vi "FindValueFromParameterNameList.vi"(10 "String":string, 11 "Matlab Param Data":T1[](array[typedef])) -> (2 "found?":bool, 3 "Matlab Data Bundle":T1)   [LabVIEW 2017]
uses:
  Types/MatlabDataBundle.ctl
  Types/MatlabDataType.ctl
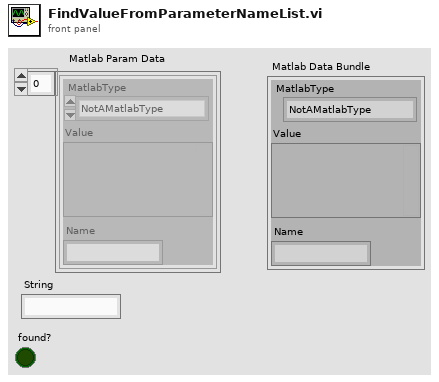
[diagram p1: front panel]
types:
  T1 = typedef "MatlabDataBundle.ctl" = cluster{"MatlabType":T2, "Value":variant, "Name":string}
  T2 = typedef "MatlabDataType.ctl" = enum16{"NotAMatlabType", "Real", "Complex", "Real Matrix", "Complex Matrix", "String", "Boolean"}
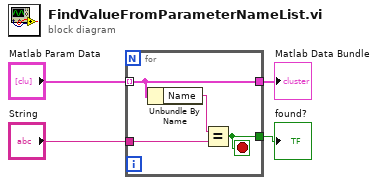
[diagram p0: block diagram]
diagram:
  n1 = for {
    tunnel: "Matlab Param Data" -> [w5] mode=indexing
    tunnel: "String" -> [w7]
    tunnel: [w6] -> w3
    tunnel: [w5] -> w2
    stop <- w6 stop-if-true
    n2 = Unbundle By Name(w5) -> ("Name"=w8:string)
    n3 = Equal?(x=w8, y=w7) -> (x = y?=w6:bool)
  }
  "found?" <- w3
  "Matlab Data Bundle" <- w2
